vi "Read RH.vi"(8 "error in (no error)":errorcluster, 11 "Vaisala Data in":refnum<class "Vaisala Data.lvclass">) -> (0 "error out":errorcluster, 2 "RH":dbl, 3 "Vaisala Data out":refnum<class "Vaisala Data.lvclass">)   [LabVIEW 2014, in "Vaisala Library.lvlib" / "Vaisala Data.lvclass"]
uses:
  Vaisala Data.lvclass
  Vaisala Data.lvclass/Vaisala Data.ctl
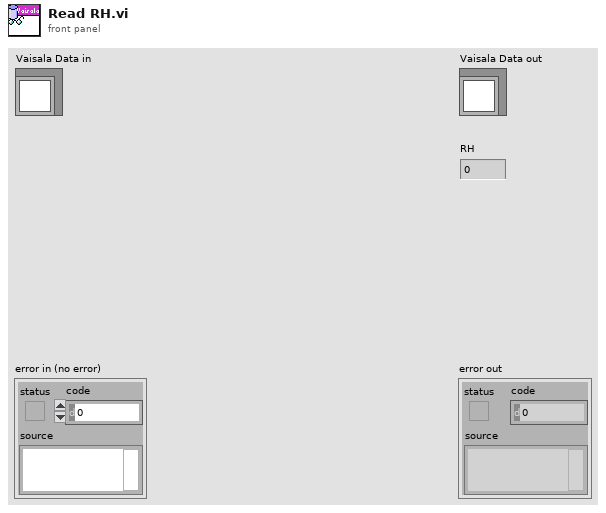
[diagram p1: front panel]
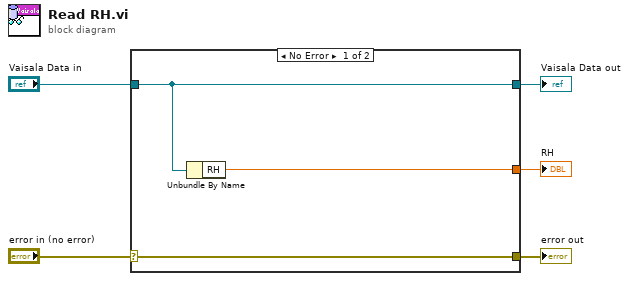
[diagram p0: block diagram]
diagram:
  n1 = case shown="No Error" "error in (no error)" {
    selector: "error in (no error)" -> [w8 w9]
    tunnel: [w8 w9] -> w4
    tunnel: [w7 w10] -> w2
    tunnel: "Vaisala Data in" -> [w7 w10]
    tunnel: [w6 _] -> w1
    frame No Error {
      n2 = Unbundle By Name(w7) -> ("RH"=w6:dbl)
    }
    frame Error {
    }
  }
  "error out" <- w4
  "Vaisala Data out" <- w2
  "RH" <- w1
